vi "command engine send commands.vi"(8 "error in (no error)":errorcluster, 9 "State Variables":T1, 10 "Settings":T4 {"Compiled"."External Channels"."Channels" format="%.0x"; "Compiled"."External Channels"."Triggers" format="%.0x"}, 11 "Global Variables":T17) -> (0 "error out":errorcluster, 1 "State Variables out":T1, 2 "Settings out":T4 {"Compiled"."External Channels"."Channels" format="%.0x"; "Compiled"."External Channels"."Triggers" format="%.0x"}, 3 "Global Variables out":T17)   [LabVIEW 2018, in "Instrument Addon Engine.lvlib"]
uses:
  Instrument Addon Engine.lvlib
  Types/Engine State Variables.ctl
  <vilib>/NI/NI VeriStand Addon Network Comm/Engine/VeriStand Comm.lvclass
  <vilib>/NI/NIVS Inline Async API/_VS Inline Async API/Process/Process.lvclass
  <vilib>/NI/NIVS Inline Async API/_Data Access Engine/Data Access Engine/Types/Write.DVR.ctl
  <vilib>/NI/NIVS Inline Async API/_Data Access Engine/Access Type Classes/Write/Write.lvclass
  <vilib>/NI/NIVS Inline Async API/_Data Access Engine/Data Access Engine/Types/Read.DVR.ctl
  <vilib>/NI/NIVS Inline Async API/_Data Access Engine/Access Type Classes/Read/Read.lvclass
  <vilib>/NI/NIVS Inline Async API/_Data Access Engine/Data Access Engine/Types/ReadWrite.DVR.ctl
  <vilib>/NI/NIVS Inline Async API/_Data Access Engine/Access Type Classes/ReadWrite/ReadWrite.lvclass
  Types/command engine global variables.ctl
  <vilib>/NI/AMC/Message Queue.ctl
  <vilib>/NI/AMC/Message.ctl
  <vilib>/NI/Tools/Keyed Array/KeyedArray.ctl
  Types/Commands RT Configuration Cluster.ctl
  Support Libraries/Protocols.lvlibp/Protocol Parent/Protocol Parent.lvclass
  Addon Shared/Types/Compiled Settings.ctl
  Addon Shared/Types/Command Parameters.ctl
  Addon Shared/Types/Linked Channel Cluster.ctl
  Addon Shared/Types/Command Channel Indeces.ctl
  Addon Shared/Types/Command Channel Index.ctl
  Addon Shared/Types/Response RT Configuration Cluster.ctl
  Addon Shared/Types/Response Parameters.ctl
  Addon Shared/Types/Response Wait Type.ctl
  Addon Shared/Types/Message Parameters.ctl
  Addon Shared/Types/Message Generation Type.ctl
  Addon Shared/Types/External Trigger Refs.ctl
  <vilib>/NI Veristand/Custom Device API/Data Reference.ctl
  Support Libraries/Protections.lvlibp/Parent Protection/Protection.lvclass
  Format Numeric to String.vi
  <vilib>/NI/Tools/Keyed Array/Tools_KeyedArray.lvlib
  <vilib>/NI/AMC/AMC.lvlib
  Addon Shared/Instrument Addon Shared.lvlib
  <vilib>/NI Veristand/Custom Device API/Custom Device API.lvlib
  <vilib>/NI/NIVS Inline Async API/_Data Access Engine/Data Access Engine/Data Access Engine.lvclass
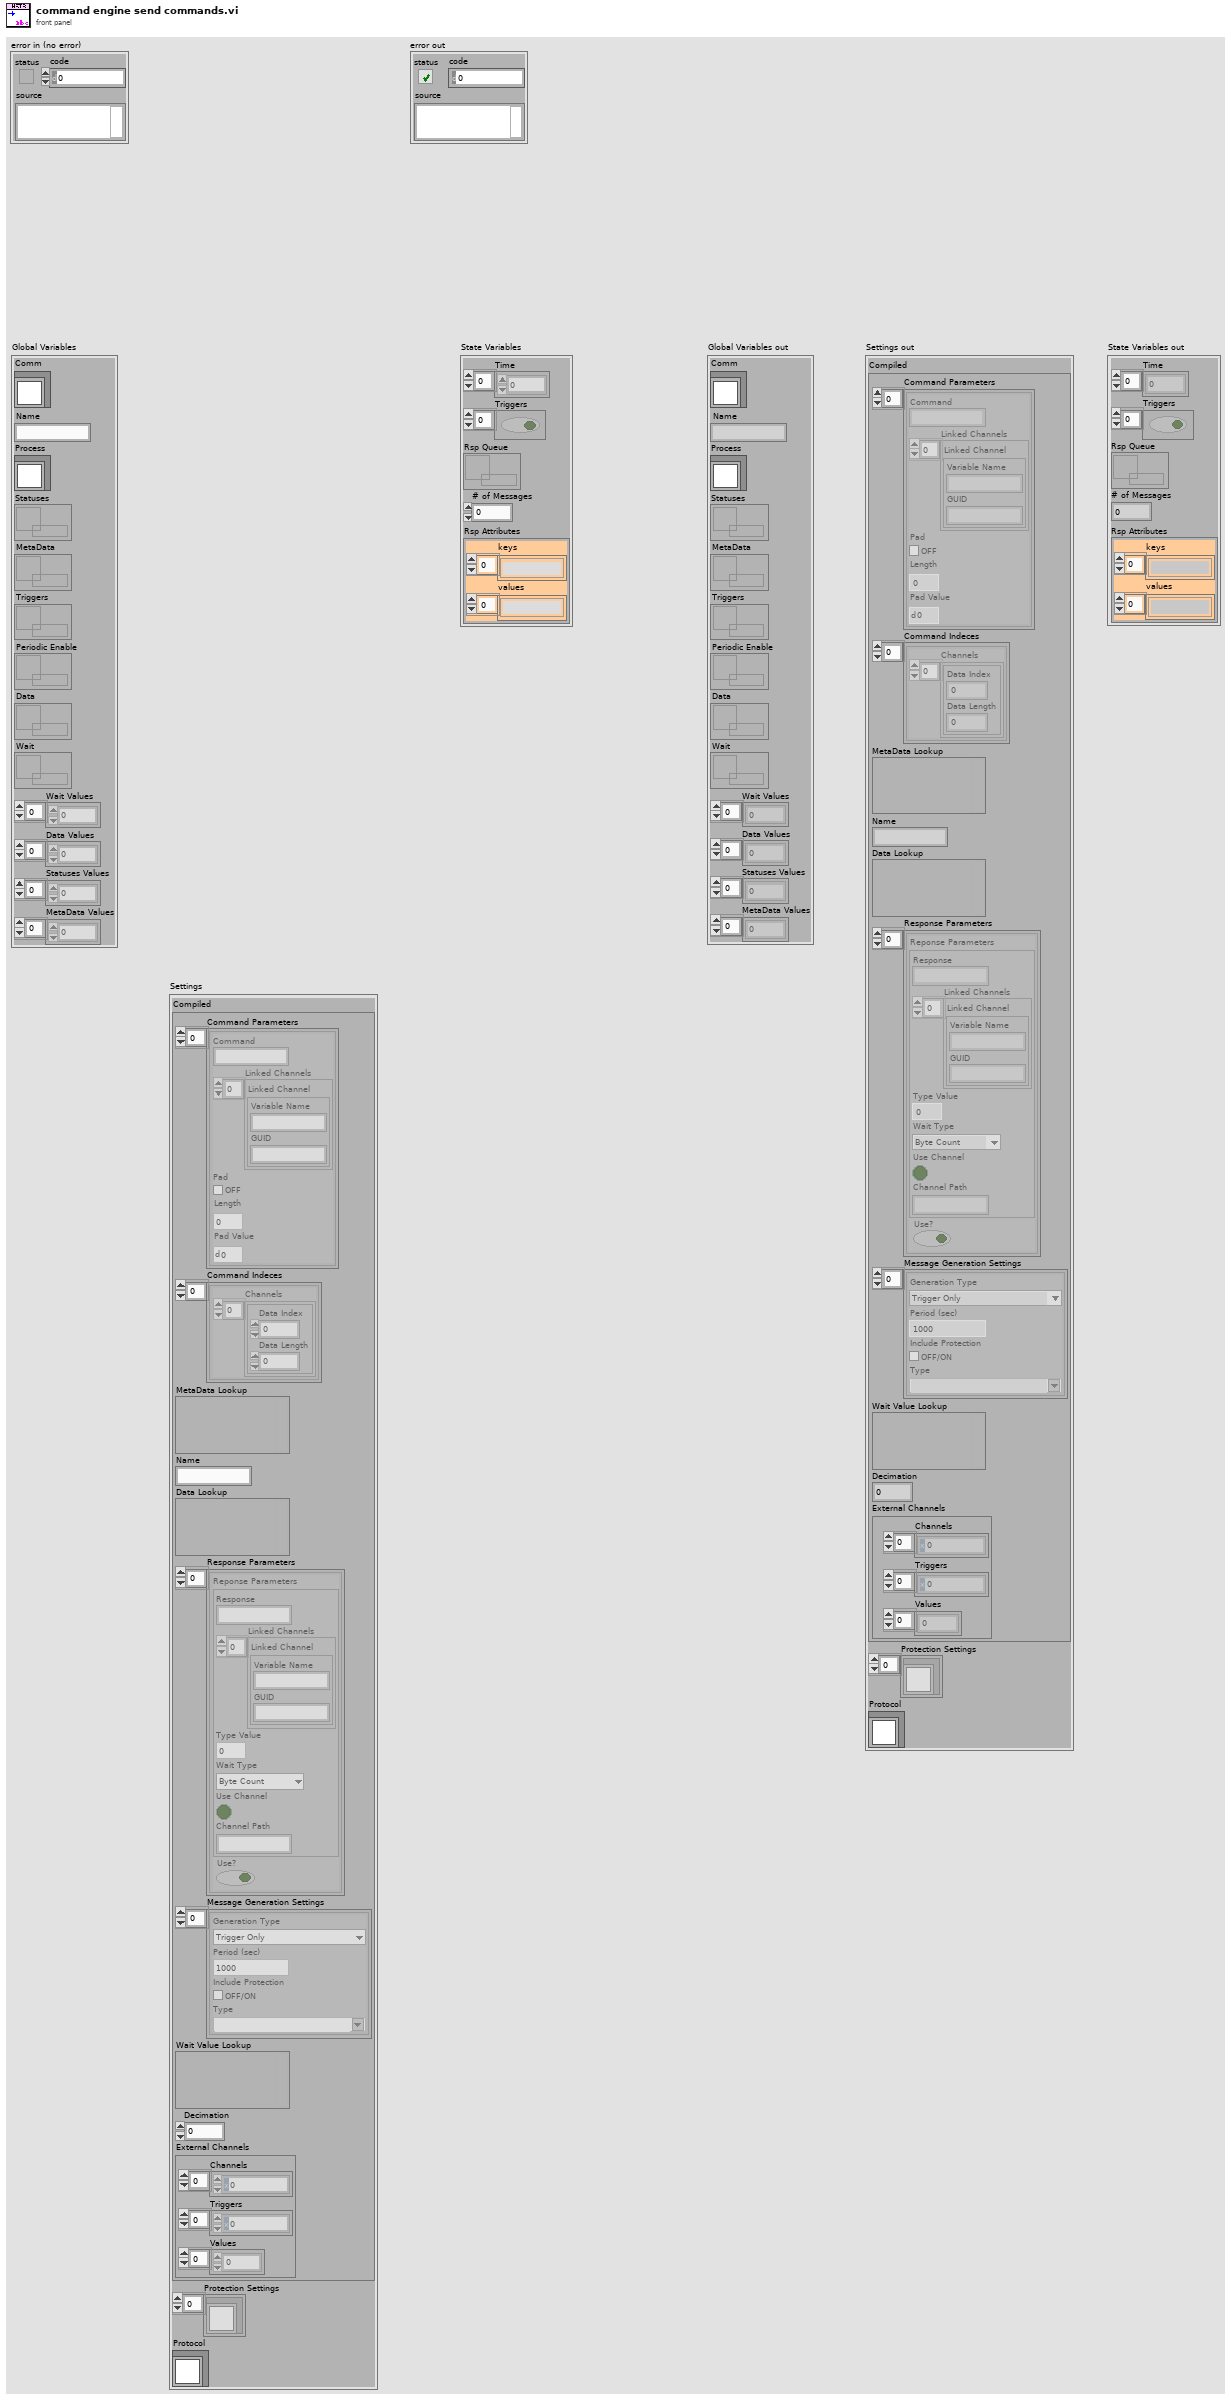
[diagram p1: front panel]
types:
  T1 = typedef "Instrument Addon Engine.lvlib/command engine global variables.ctl" = cluster{"Time":u32[], "Triggers":bool[], "Rsp Queue":T2, "# of Messages":i32, "Rsp Attributes":T3}
  T2 = typedef "AMC.lvlib/Message Queue.ctl" = refnum<queue>
  T3 = typedef "Tools_KeyedArray.lvlib/KeyedArray.ctl" = cluster{"keys":string[], "values":string[]}
  T4 = typedef "Instrument Addon Engine.lvlib/Commands RT Configuration Cluster.ctl" = cluster{"Compiled":T5, "Protection Settings":refnum<class "Protection.lvclass">[], "Protocol":refnum<class "Protocol Parent.lvclass">}
  T5 = typedef "Instrument Addon Shared.lvlib/Compiled Settings.ctl" = cluster{"Command Parameters":T6[], "Command Indeces":T8[], "MetaData Lookup":variant, "Name":string, "Data Lookup":variant, "Response Parameters":T10[], "Message Generation Settings":T13[], "Wait Value Lookup":variant, "Decimation":u32, "External Channels":T15}
  T6 = typedef "Instrument Addon Shared.lvlib/Command Parameters.ctl" = cluster{"Command":string, "Linked Channels":T7[], "Pad":bool, "Length":u32, "Pad Value":u8}
  T7 = typedef "Instrument Addon Shared.lvlib/Linked Channel Cluster.ctl" = cluster{"Variable Name":string, "GUID":string}
  T8 = typedef "Instrument Addon Shared.lvlib/Command Channel Indeces.ctl" = cluster{"Channels":T9[]}
  T9 = typedef "Instrument Addon Shared.lvlib/Command Channel Index.ctl" = cluster{"Data Index":i32, "Data Length":i32}
  T10 = typedef "Instrument Addon Shared.lvlib/Response RT Configuration Cluster.ctl" = cluster{"Reponse Parameters":T11, "Use?":bool}
  T11 = typedef "Instrument Addon Shared.lvlib/Response Parameters.ctl" = cluster{"Response":string, "Linked Channels":T7[], "Type Value":dbl, "Wait Type":T12, "Use Channel":bool, "Channel Path":string}
  T12 = typedef "Instrument Addon Shared.lvlib/Response Wait Type.ctl" = enum16{"Byte Count", "Wait sec"}
  T13 = typedef "Instrument Addon Shared.lvlib/Message Parameters.ctl" = cluster{"Generation Type":T14, "Period":dbl, "Include Protection":bool, "Type":string}
  T14 = typedef "Instrument Addon Shared.lvlib/Message Generation Type.ctl" = enum16{"Trigger Only", "Periodic & Trigger", "Value Change & Trigger"}
  T15 = typedef "Instrument Addon Shared.lvlib/External Trigger Refs.ctl" = cluster{"Channels":T16[], "Triggers":T16[], "Values":dbl[]}
  T16 = typedef "Custom Device API.lvlib/Data Reference.ctl" = i32
  T17 = typedef "Instrument Addon Engine.lvlib/Engine State Variables.ctl" = cluster{"Comm":refnum<class "VeriStand Comm.lvclass">, "Name":string, "Process":refnum<class "Process.lvclass">, "Statuses":T18, "MetaData":T19, "Triggers":T20, "Periodic Enable":T19, "Data":T18, "Wait":T19, "Wait Values":dbl[], "Data Values":dbl[], "Statuses Values":dbl[], "MetaData Values":dbl[]}
  T18 = typedef "Data Access Engine.lvlib/Data Access Engine.lvclass/Write.DVR.ctl" = refnum<data-value>
  T19 = typedef "Data Access Engine.lvlib/Data Access Engine.lvclass/Read.DVR.ctl" = refnum<data-value>
  T20 = typedef "Data Access Engine.lvlib/Data Access Engine.lvclass/ReadWrite.DVR.ctl" = refnum<data-value>
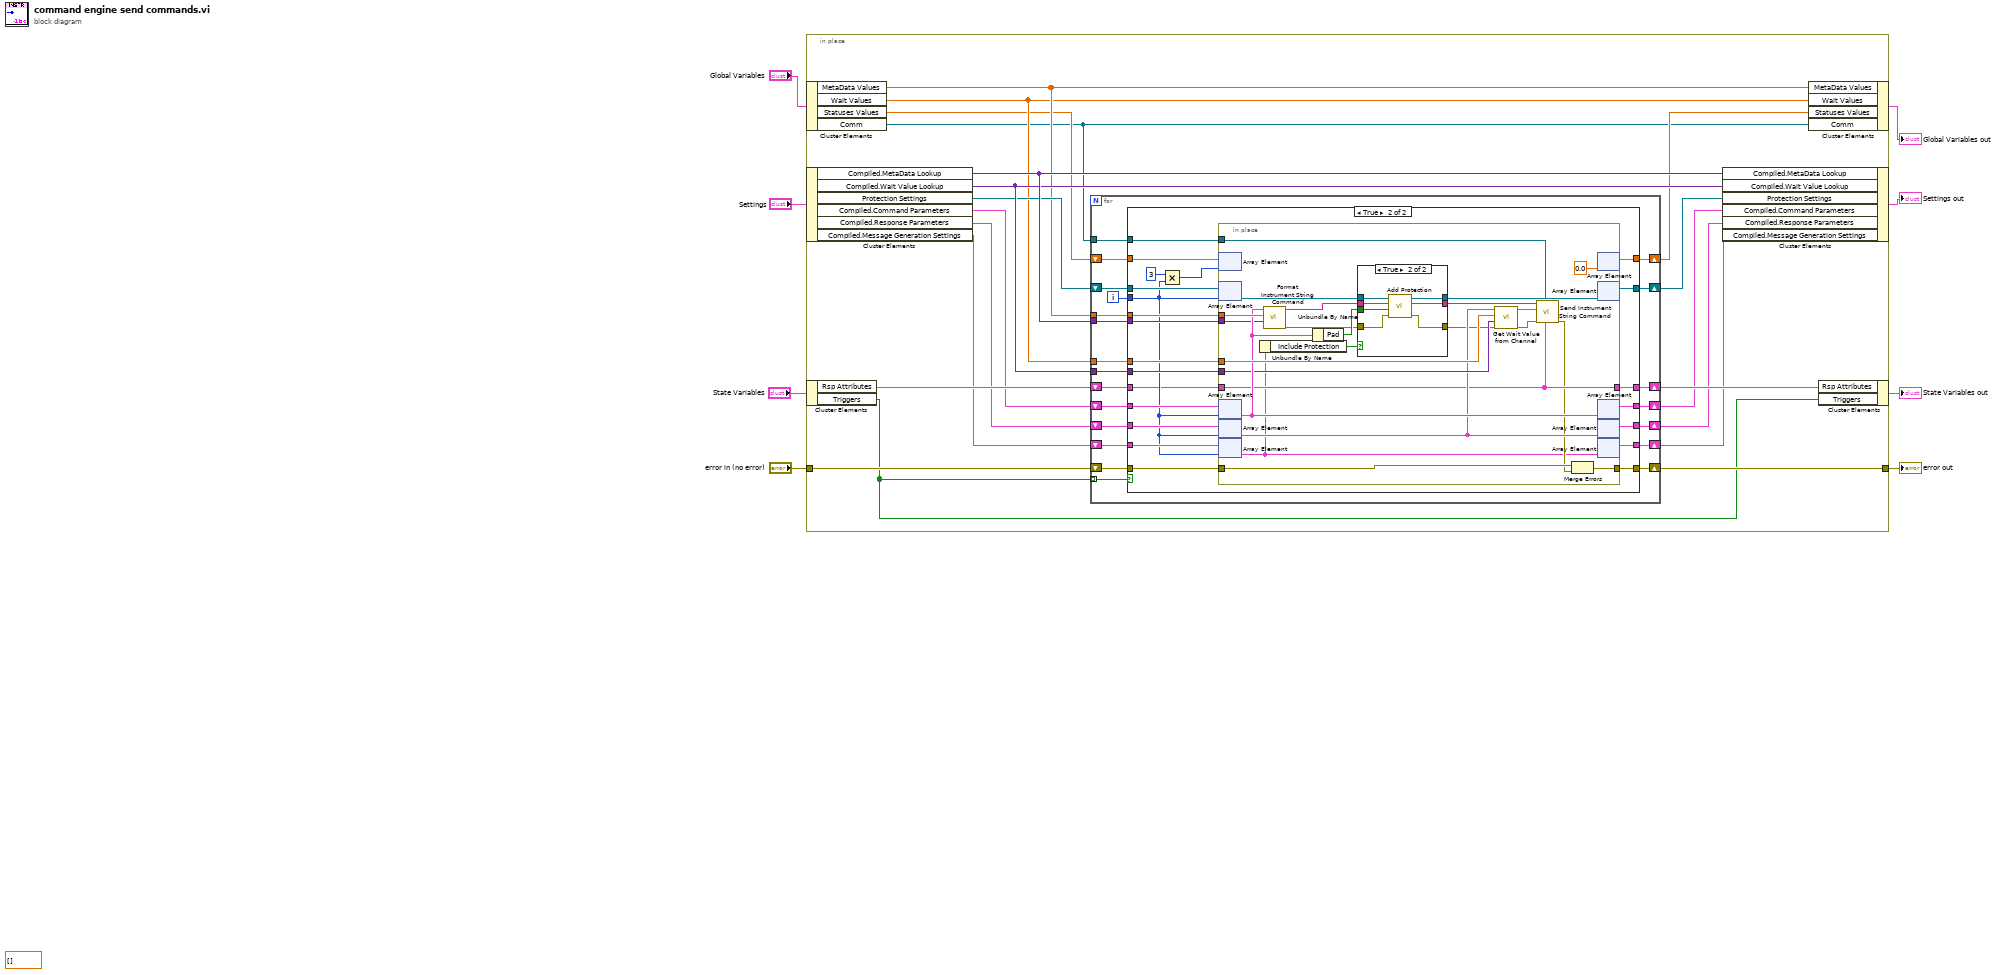
[diagram p0: block diagram]
diagram:
  (unwired) dbl[] []
  n1 = in-place {
    in-place-border: "error in (no error)" -> [w28]
    in-place-border: [w17] -> w4
    n2 = in-place-cluster #1("Global Variables") -> ("MetaData Values"=w13:dbl[], "Wait Values"=w12:dbl[], "Statuses Values"=w10:dbl[], "Comm"=w9:refnum<class "VeriStand Comm.lvclass">)
    n3 = in-place-cluster #2("Settings") -> ("Compiled.MetaData Lookup"=w27:variant, "Compiled.Wait Value Lookup"=w26:variant, "Protection Settings"=w16:refnum<class "Protection.lvclass">[], "Compiled.Command Parameters"=w19:T6[], "Compiled.Response Parameters"=w21:T10[], "Compiled.Message Generation Settings"=w23:T13[])
    n4 = in-place-cluster #3("State Variables") -> ("Rsp Attributes"=w25:T3, "Triggers"=w14:bool[])
    n5 = for {
      shift-right: [w41] -> w11
      shift-left: w10 -> [w42]
      shift-right: [w43] -> w20
      shift-left: w21 -> [w44]
      shift-right: [w39] -> w22
      shift-left: w23 -> [w40]
      shift-right: [w45] -> w15
      shift-left: w16 -> [w46]
      shift-right: [w30] -> w24
      shift-left: w25 -> [w31]
      shift-right: [w37] -> w18
      shift-left: w19 -> [w38]
      tunnel: w26 -> [w47]
      tunnel: w27 -> [w36]
      tunnel: w12 -> [w35]
      tunnel: w13 -> [w34]
      tunnel: w9 -> [w33]
      shift-right: [w48] -> w17
      shift-left: w28 -> [w49]
      tunnel: w14 -> [w29] mode=indexing
      i -> [w32]
      n6 = case shown="True" w29 {
        tunnel: w49 -> [w54 w78]
        tunnel: [w54 w77] -> w48
        tunnel: w47 -> [_ w76]
        tunnel: w46 -> [w55 w75]
        tunnel: [w55 w74] -> w45
        tunnel: w44 -> [w51 w73]
        tunnel: [w51 w72] -> w43
        tunnel: w42 -> [w56 w71]
        tunnel: [w56 w68] -> w41
        tunnel: w40 -> [w50 w67]
        tunnel: [w50 w66] -> w39
        tunnel: w38 -> [w52 w65]
        tunnel: [w52 w64] -> w37
        tunnel: w36 -> [_ w63]
        tunnel: w35 -> [_ w62]
        tunnel: w34 -> [_ w61]
        tunnel: w33 -> [_ w60]
        tunnel: w32 -> [_ w59]
        tunnel: w31 -> [w53 w58]
        tunnel: [w53 w57] -> w30
        frame False {
        }
        frame True {
          n7 = Multiply(x=3, y=w59) -> (x*y=w69:i32)
          n8 = in-place {
            in-place-border: w78 -> [w101]
            in-place-border: [w100] -> w77
            in-place-border: w61 -> [w93]
            in-place-border: w63 -> [w90]
            in-place-border: w76 -> [w91]
            in-place-border: w62 -> [w94]
            in-place-border: w60 -> [w79]
            in-place-border: w58 -> [w88]
            in-place-border: [w88] -> w57
            n9 = in-place-array #4(w71, w69) -> ()  [unwired: 1 out]
            n10 = in-place-array #5(w75, w59) -> (w97:refnum<class "Protection.lvclass">)
            n11 = in-place-array #6(w65, w59) -> (w92:T6)
            n12 = in-place-array #7(w73, w59) -> (w89:T10)
            n13 = in-place-array #8(w67, w59) -> (w80:T13)
            n14 = Unbundle By Name(w80) -> ("Include Protection"=w98:bool)
            n15 = call "Format Instrument String Command.vi"("MetaData Lookup in"=w90, "MetaData"=w93, "Command Parameters"=w92) -> ("error out"=w83:errorcluster, "Command"=w84:string)  [unwired: 6 in, 1 out]
            n16 = Unbundle By Name(w92) -> ("Pad"=w99:bool)
            n17 = case shown="True" w98 {
              tunnel: w84 -> [w103 w111]
              tunnel: w83 -> [w104 w110]
              tunnel: [w104 w109] -> w82
              tunnel: [w103 w108] -> w81
              tunnel: w99 -> [_ w107]
              tunnel: w97 -> [w102 w106]
              tunnel: [w102 w105] -> w96
              frame False {
              }
              frame True {
                n18 = call-dynamic "Add Protection.vi"("error in (no error)"=w110, "Pad"=w107, "String in"=w111, "Protection in"=w106) -> ("error out"=w109:errorcluster, "String out"=w108:string, "Protection out"=w105:refnum<class "Protection.lvclass">)  [unwired: 5 in]
              }
            }
            n19 = call "Get Wait Value from Channel.vi"("error in (no error)"=w82, "Wait Value Lookup"=w91, "Wait Values"=w94, "Response"=w89) -> ("error out"=w85:errorcluster, "Response out"=w86:T10)  [unwired: 6 in]
            n20 = call "Send Instrument String Command.vi"("message attributes"=w88, "Comm"=w79, "error in (no error)"=w85, "Response Parameters"=w86, "Command"=w81) -> ("error out"=w87:errorcluster)  [unwired: 6 in]
            n21 = Merge Errors(w101, w87) -> (w100:errorcluster)
            n22 = in-place-array #4(0.0) -> (w68:dbl[])  [unwired: 1 out]
            n23 = in-place-array #5(w96) -> (w74:refnum<class "Protection.lvclass">[])  [unwired: 1 out]
            n24 = in-place-array #6(w92) -> (w64:T6[])  [unwired: 1 out]
            n25 = in-place-array #7(w89) -> (w72:T10[])  [unwired: 1 out]
            n26 = in-place-array #8(w80) -> (w66:T13[])  [unwired: 1 out]
          }
        }
      }
    }
    n27 = in-place-cluster #2("Compiled.MetaData Lookup"=w27, "Compiled.Wait Value Lookup"=w26, "Protection Settings"=w15, "Compiled.Command Parameters"=w18, "Compiled.Response Parameters"=w20, "Compiled.Message Generation Settings"=w22) -> (→"Settings out":T4)
    n28 = in-place-cluster #1("MetaData Values"=w13, "Wait Values"=w12, "Statuses Values"=w11, "Comm"=w9) -> (→"Global Variables out":T17)
    n29 = in-place-cluster #3("Rsp Attributes"=w24, "Triggers"=w14) -> (→"State Variables out":T1)
  }
  "error out" <- w4
